vi "HasErrors.vi"(8 "error in (no error)":errorcluster, 11 "ErrorManager in":refnum<class "ErrorManager.lvclass">) -> (0 "error out":errorcluster, 1 "empty?":bool, 3 "ErrorManager out":refnum<class "ErrorManager.lvclass">)   [LabVIEW 2020, in "ErrorManager.lvlib" / "ErrorManager.lvclass"]
uses:
  ErrorManager.lvclass
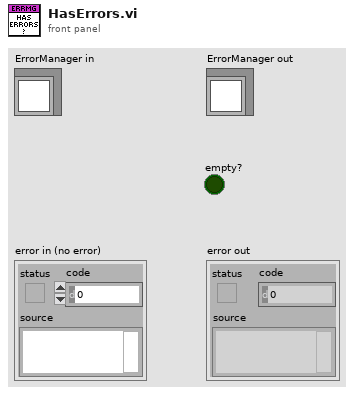
[diagram p1: front panel]
types:
  T1 = typedef "ErrorManager.lvlib/ErrorManager.lvclass/ErrorInfoArrayRef.ctl" = refnum<data-value>
  T2 = typedef "ErrorManager.lvlib/ErrorManager.lvclass/ErrorInfo.ctl" = cluster{"Time Stamp":timestamp, "Message":string, "Type":T3}
  T3 = typedef "LabVIEWObjectInterfaces.lvlib/IErrorManager.lvclass/ErrorType.ctl" = enum16{"Info", "Warning", "Error"}
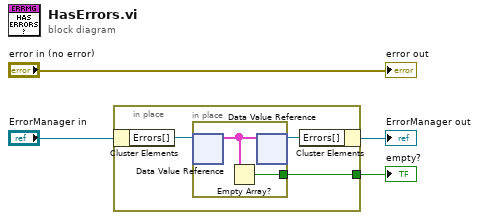
[diagram p0: block diagram]
diagram:
  n1 = in-place {
    in-place-border: [w6] -> w2
    n2 = in-place-cluster #1("ErrorManager in") -> ("Errors[]"=w7:T1)
    n3 = in-place {
      in-place-border: [w8] -> w6
      n4 = in-place-dvr #2(w7) -> (w9:T2[])  [unwired: 1 out]
      n5 = Empty Array?(array=w9) -> (empty?=w8:bool)
      n6 = in-place-dvr #2(w9) -> (w5:T1)  [unwired: 1 out]
    }
    n7 = in-place-cluster #1("Errors[]"=w5) -> (→"ErrorManager out":refnum<class "ErrorManager.lvclass">)
  }
  "empty?" <- w2
  "error out" <- "error in (no error)"
